vi "Byte36_39 (SubVI).vi"(1 "Input String":string) -> (0 "UTC Time":timestamp)   [LabVIEW 2024]
panel:
  out "UTC Time LSW":u16
  out "UTC Time MSW":u16
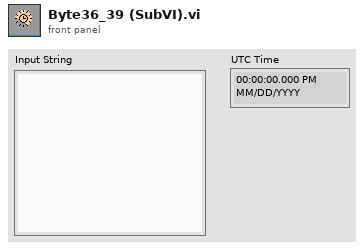
[diagram p1: front panel]
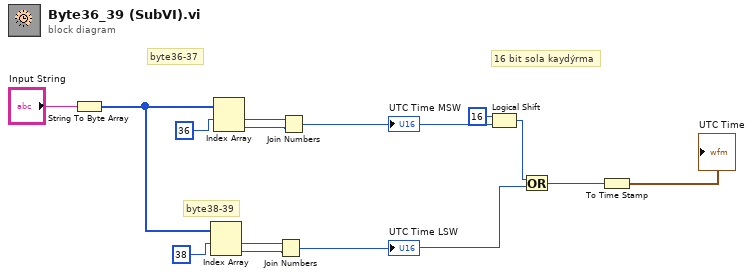
[diagram p0: block diagram]
diagram:
  # "16 bit sola kaydýrma"
  # "byte38-39"
  # "byte36-37"
  n1 = String To Byte Array(string="Input String") -> (unsigned byte array=w7:u8[])
  n2 = Index Array "Index Array"(array=w7, index #1=38 ("index")) -> (element #1=w9:u8, element #2=w8:u8)  [unwired: 1 in]
  n3 = Index Array "Index Array"(array=w7, index #1=36 ("index")) -> (element #1=w12:u8, element #2=w11:u8)  [unwired: 1 in]
  n4 = Join Numbers(hi=w9, lo=w8) -> ((hi.lo)=w4:u16)
  "UTC Time LSW" <- w4
  n5 = Join Numbers(hi=w12, lo=w11) -> ((hi.lo)=w6:u16)
  "UTC Time MSW" <- w6
  n6 = Logical Shift(y=i16 16, x=w6) -> (x << y=w3:u16)
  n7 = Or(x=w3, y=w4) -> (x .or. y?=w2:u16)
  n8 = To Time Stamp(1:w2) -> (0:→"UTC Time":timestamp)
